vi "Disable XBox Drive & Steer.vi"   [LabVIEW 2011]
uses:
  _GlobalVariables&Libraries/ATV Program Global Variables.vi
types:
  T1 = cluster{"Drive Value Output String":string, "Steer Value Output String":string, "Button A":bool, "Button B":bool, "Error Out":errorcluster, "Disable XBox Drive & Steer":bool, "Disable XBox Controller":bool, "XBOX Button Trigger Time (ms)":u32, "Button X":bool, "Button Y":bool}
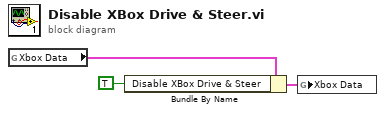
[diagram p0: block diagram]
diagram:
  n1 = global read "ATV Program Global Variables.vi" "Xbox Data"() -> (w1:T1)
  n2 = Bundle By Name(cluster=w1, "Disable XBox Drive & Steer"=TRUE) -> (w2:T1)
  n3 = global write "ATV Program Global Variables.vi" "Xbox Data"(w2) -> ()
